vi "Get Message.vi"(8 "error in (no error)":errorcluster, 11 "Message Transport Singleton in":refnum<class "Message Transport Singleton.lvclass">=refnum) -> (0 "error out":errorcluster, 3 "Message":refnum<class "Message Interface.lvclass">)   [LabVIEW 2016, in "Stream Mediator.lvlib" / "Message Transport Singleton.lvclass"]
doc: "--\nCopyright © 2017 Composed SystemsI All rights reserved.\n\nAuthor: Jon McBee <jon.mcbee@composed.io>\n\nThis library is provided \"AS IS\" ,WITHOUT WARRANTIES OR\nCONDITIONS OF ANY KIND, either express or implied.\n\nComposed Systems -- composed.io\n\nStream 0.0.1.1\nJon McBee - Composed Systems\nCopyright (c) 2017, Composed Systems"
uses:
  <userlib>/Composed Systems/Stream/Mediator/Classes/Message Transport Singleton/Message Transport Singleton.lvclass
  <userlib>/Composed Systems/Stream/Mediator/Classes/Message Interface/Message Interface.lvclass
  <userlib>/Composed Systems/Stream/Mediator/Classes/Message Transport Singleton/Message Transport Singleton.lvclass/Message Transport Singleton.ctl
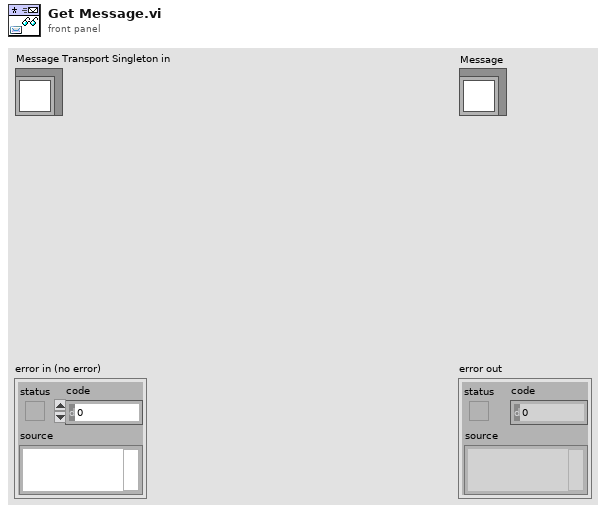
[diagram p1: front panel]
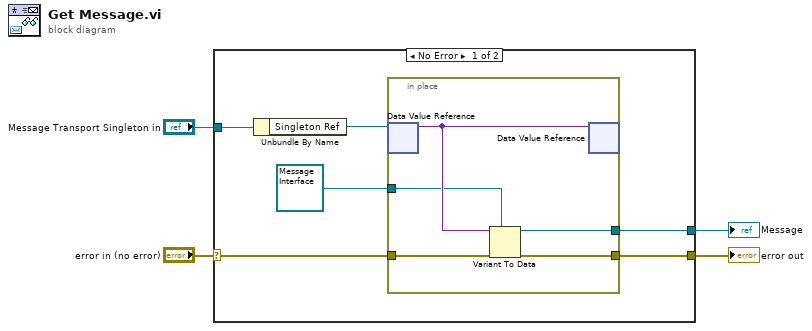
[diagram p0: block diagram]
diagram:
  n1 = case shown="No Error" "error in (no error)" {
    selector: "error in (no error)" -> [w8 w16]
    tunnel: [w7 w16] -> w3
    tunnel: "Message Transport Singleton in" -> [w10 _]
    tunnel: [w5 _] -> w1
    frame No Error {
      n2 = Unbundle By Name(w10) -> ("Singleton Ref"=w9:refnum<data-value>)
      n3 = in-place {
        in-place-border: [w13] -> w7
        in-place-border: w8 -> [w14]
        in-place-border: refnum<class "Message Interface.lvclass"> refnum ("Stream Mediator.lvlib:Message Interface.lvclass") -> [w12]
        in-place-border: [w11] -> w5
        n4 = in-place-dvr #1(w9) -> (w15:variant)  [unwired: 1 out]
        n5 = Variant To Data(error in=w14, type=w12, Variant=w15) -> (data=w11:refnum<class "Message Interface.lvclass">, error out=w13:errorcluster)
        n6 = in-place-dvr #1(w15) -> ()  [unwired: 2 out]
      }
    }
    frame Error {
    }
  }
  "error out" <- w3
  "Message" <- w1
